vi "12.2-5 Reject Border.vi"() -> ()   [LabVIEW 2016]
doc: "This example shows how to use the Edge Tool in NI Vision. The Edge Tool finds edges (or sharp transitions in the pixels values) along a given line or ROI profile. The Edge Tool is a precursor function to many of the gauging and inspection tasks. For example, the location of the edges found along a line profile across an object can interpreted as the boundaries of the object whose dimensions have to be measured for a gauging application or the presence of a crack in the surface of an object for an inspection application."
uses:
  <vilib>/vision/NI_Vision_Development_Module.lvlib
panel:
  out "Dst":T1(plugin-control) caption="Results"
  out "Src":T1(plugin-control) caption="Source Image"
  in  "Connectivity 4/8 (8)":bool=TRUE
  in  "Structuring Element":i32[][](array[numeric])=[[0, 1, 0], [1, 1, 1], [0, 0, 0]]
  in  "Hexa Pixel?":bool
  in  "# of iterations":i32=1
  in  "Operation":u16(ring) items=["AutoM", "Close", "Dilate", "Erode", "Gradient", "Gradient out", "Gradient in", "Hit miss", "Open", "PClose", "POpen", "Thick", "Thin"]
  in  "Stop":bool
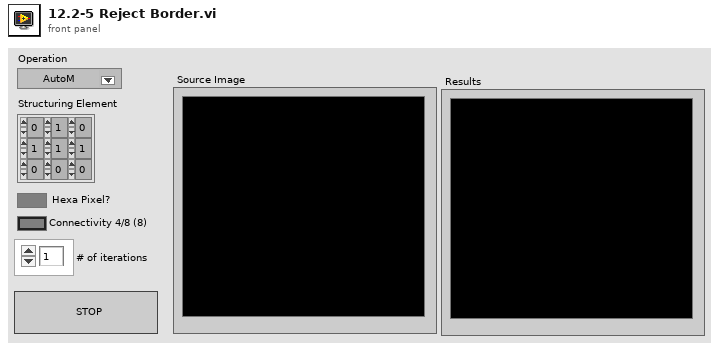
[diagram p1: front panel]
types:
  T1 = typedef "IMAQ Image.ctl" = refnum<image>
  T2 = cluster{"Hexa Pixel?":bool, "Operation":u16, "Structuring Element":i32[][], "# of iterations":i32, "Connectivity 4/8 (8)":bool}
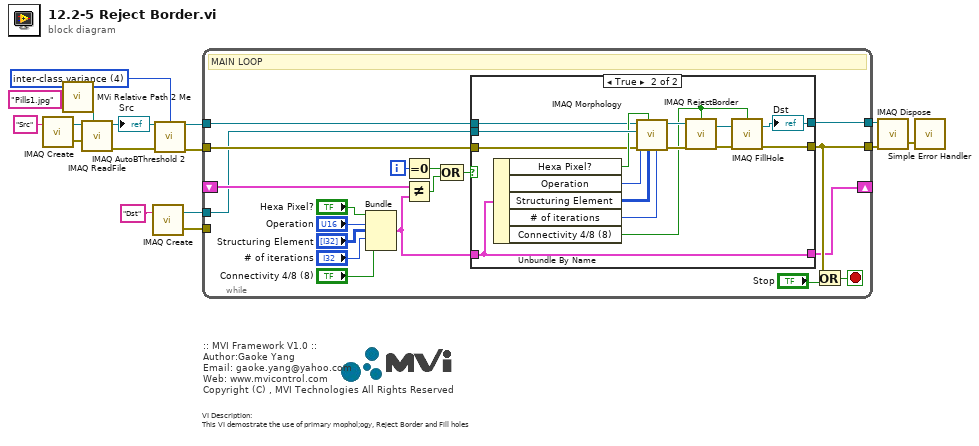
[diagram p0: block diagram]
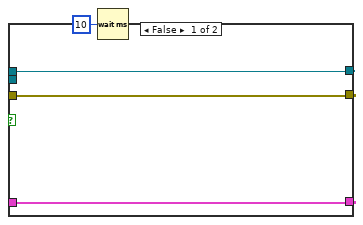
[diagram p2: hidden frame]
diagram:
  w5 = 4 items=["clustering", "entropy", "metric", "moments", "inter-class variance"] ("Method")
  # "VI Description:\nThis VI demostrate the use of primary mophol;ogy, Reject Border and Fill holes"
  # ":: MVI Framework V1.0 ::\nAuthor:Gaoke Yang\nEmail: gaoke.yang@yahoo.com\nWeb: www.mvicontrol.com\nCopyright (C) , MVI Technologies All Rights Reserved"
  n1 = call "IMAQ Create"("Image Name"="Src") -> ("New Image"=w15:T1, "error out"=w14:errorcluster)  [unwired: 4 in]
  n2 = call "MVi Relative Path 2 Me.vi"("Relative Path"="Pills1.jpg" ("name or relative path")) -> ("Appended Dir"=w10:path)  [unwired: 5 in, 1 out]
  n3 = call "IMAQ ReadFile"("File Path"=w10, "error in (no error)"=w14, "Image"=w15) -> ("error out"=w2:errorcluster, "Image Out"=w1:T1)  [unwired: 4 in, 3 out]
  "Src" <- w1
  n4 = call "IMAQ Create"("Image Name"="Dst") -> ("New Image"=w7:T1, "error out"=w6:errorcluster)  [unwired: 4 in]
  n5 = call "IMAQ AutoBThreshold 2"("Image Src"=w1, "Method (clustering)"=w5, "error in (no error)"=w2) -> ("Image Dst Out"=w3:T1, "error out"=w4:errorcluster)  [unwired: 5 in, 6 out]
  n6 = while "MAIN LOOP" {
    tunnel: w3 -> [w34]
    tunnel: w4 -> [w35]
    tunnel: [w30] -> w13
    tunnel: [w31] -> w12
    shift-right: [w27] -> _
    shift-left: _ -> [w24]
    tunnel: w7 -> [w22]
    tunnel: w6 -> [_]
    i -> [w29]
    stop <- w32 stop-if-true
    # "MAIN LOOP"
    n7 = Bundle("Hexa Pixel?"="Hexa Pixel?", "Operation"="Operation", "Structuring Element"="Structuring Element", "# of iterations"="# of iterations", "Connectivity 4/8 (8)"="Connectivity 4/8 (8)") -> (w25:T2)  [unwired: 1 in]
    n8 = Equal To 0?(x=w29) -> (x = 0?=w26:bool)
    n9 = Not Equal?(x=w24, y=w25) -> (x != y?=w23:bool)
    n10 = Compound Arithmetic op=OR(w26, w23) -> (w28:bool)
    n11 = case shown="True" w28 {
      tunnel: w35 -> [w38 w47]
      tunnel: w34 -> [w39 w48]
      tunnel: [w39 w40] -> w31
      tunnel: [w38 w43] -> w30
      tunnel: [w36 w53] -> w27
      tunnel: w25 -> [w36 w53]
      tunnel: w22 -> [_ w54]
      frame False {
        n12 = Wait (ms)(milliseconds to wait=u32 10) -> ()  [unwired: 1 out]
      }
      frame True {
        n13 = Unbundle By Name(w53) -> ("Hexa Pixel?"=w49:bool, "Operation"=w50:u16, "Structuring Element"=w51:i32[][], "# of iterations"=w52:i32, "Connectivity 4/8 (8)"=w42:bool)
        n14 = call "IMAQ Morphology"("Number of iterations (1)"=w52, "Structuring Element"=w51, "Square/Hexa (Square)"=w49, "error in (no error)"=w47, "Operation"=w50, "Image Dst"=w54, "Image Src"=w48) -> ("error out"=w46:errorcluster, "Image Dst Out"=w45:T1)  [unwired: 3 in]
        n15 = call "IMAQ RejectBorder"("error in (no error)"=w46, "Image Src"=w45, "Connectivity 4/8 (8)"=w42) -> ("error out"=w44:errorcluster, "Image Dst Out"=w41:T1)  [unwired: 3 in]
        n16 = call "IMAQ FillHole"("error in (no error)"=w44, "Image Src"=w41, "Connectivity 4/8 (8)"=w42) -> ("error out"=w43:errorcluster, "Image Dst Out"=w40:T1)  [unwired: 3 in]
        "Dst" <- w40
      }
    }
    n17 = Or(x=w30, y="Stop") -> (x .or. y?=w32:bool)
  }
  n18 = call "IMAQ Dispose"("Image"=w12, "error in (no error)"=w13) -> ("error out"=w9:errorcluster)  [unwired: 4 in]
  n19 = call <vilib>:"Simple Error Handler.vi"("error in (no error)"=w9) -> ()  [unwired: 4 in, 5 out]
